vi "Read XML file.vi"(8 "error in (no error)":errorcluster, 11 "file path (use dialog)":path) -> (0 "error out":errorcluster, 3 "Array 3":string[](array[string]))   [LabVIEW 2012]
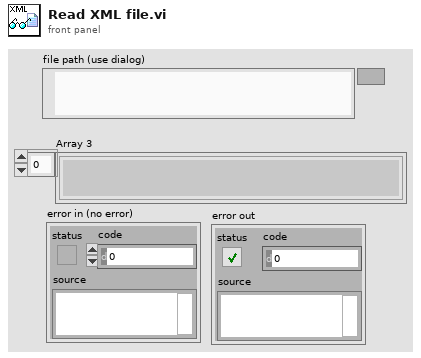
[diagram p1: front panel]
types:
  T1 = enum16{"open", "replace", "create", "open or create", "replace or create", "replace or create with confirmation"}
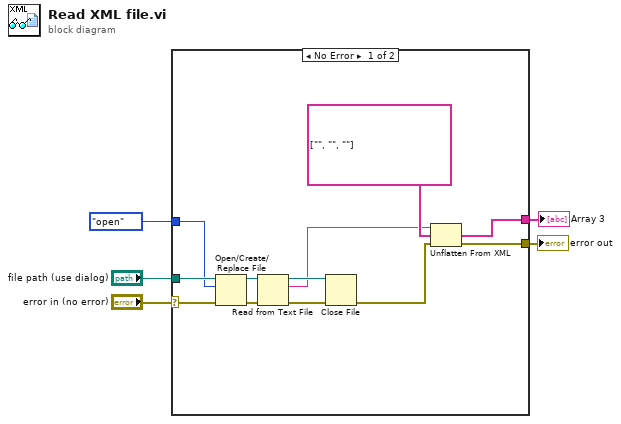
[diagram p0: block diagram]
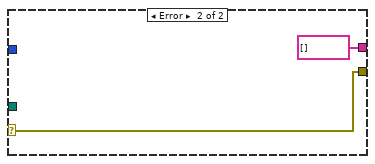
[diagram p2: hidden frame]
diagram:
  n1 = case shown="No Error" "error in (no error)" {
    selector: "error in (no error)" -> [w7 w18]
    tunnel: [w15 string[] [] ("Array 3")] -> w5
    tunnel: "file path (use dialog)" -> [w14 _]
    tunnel: T1."open" ("operation (0:open)") -> [w13 _]
    tunnel: [w8 w18] -> w2
    frame No Error {
      n2 = Open/Create/Replace File(file path (use dialog)=w14, error in=w7, operation (0:open)=w13) -> (refnum out=w11:refnum<file>, error out=w12:errorcluster)  [unwired: 3 in, 1 out]
      n3 = Read from Text File(file (use dialog)=w11, error in=w12) -> (refnum out=w17:refnum<file>, text=w6:string, error out=w10:errorcluster)  [unwired: 2 in, 1 out]
      n4 = Close File(refnum=w17, error in=w10) -> (error out=w9:errorcluster)  [unwired: 1 out]
      n5 = Unflatten From XML(xml string=w6, type=string[] ["", "", ""] ("Array 3"), error in (no error)=w9) -> (value=w15:string[], error out=w8:errorcluster)
    }
    frame Error {
    }
  }
  "error out" <- w2
  "Array 3" <- w5
